vi "Do.vi"(8 "Error In":errorcluster, 10 "Actor in":refnum<class "Actor.lvclass">, 11 "CS++LNAMessage":refnum<class "CS++LNAMessage.lvclass">) -> (0 "Error Out":errorcluster, 2 "Actor out":refnum<class "Actor.lvclass">)   [LabVIEW 2014, in "CS++LNA.lvlib" / "CS++LNAMessage.lvclass"]
doc: "This VI creates the desired message object as class default object. Derives message classes need to override the <b>Parameter to Attribute.vi</b> to parse the variant attributes to the message object attribute.\n\nVI-Parameter Names of corresponding public VI of the derived actor class = Variant Attribute Names\n\n(<B>Filename</B>: Actor Framework.lvlib:Message.lvclass:Do.vi)\n\nDefines what a message does when it is received by an actor. Generally, a message instructs an actor to invoke one of its methods. By default, this method does nothing. A child class must override it to define behavior. Create a child class by using the Actor Framework Message Maker dialog box."
uses:
  CS++LNAMessage.lvclass
  <vilib>/ActorFramework/Actor/Actor.lvclass
  <vilib>/ActorFramework/Message/Message.lvclass
  CS++LNAMessage.lvclass/CS++LNAMessage.ctl
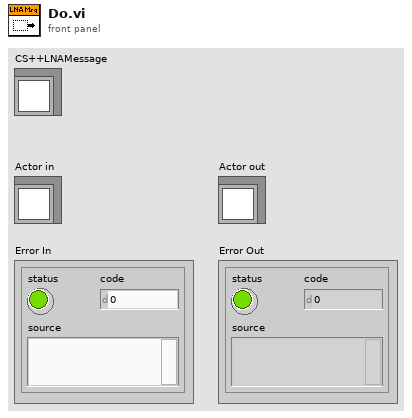
[diagram p1: front panel]
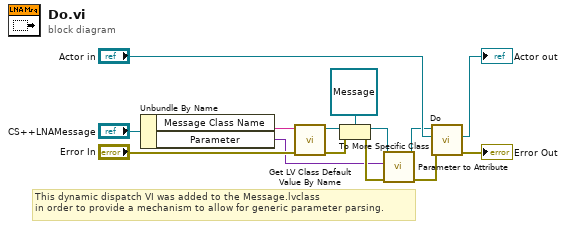
[diagram p0: block diagram]
diagram:
  # "This dynamic dispatch VI was added to the Message.lvclass\nin order to provide a mechanism to allow for generic parameter parsing."
  n1 = Unbundle By Name("CS++LNAMessage") -> ("Message Class Name"=w7:string, "Parameter"=w1:variant)
  n2 = call <vilib>:"Get LV Class Default Value By Name.vi"("error in (no error)"="Error In", "class name"=w7) -> ("error out"=w10:errorcluster, "object"=w9:refnum<class>)  [unwired: 8 in]
  n3 = To More Specific Class(target class=refnum<class "Message.lvclass"> refnum ("Message"), reference=w9, error in=w10) -> (specific class reference=w5:refnum<class "Message.lvclass">, error out=w3:errorcluster)
  n4 = call-dynamic "Parameter to Attribute.vi"("error in (no error)"=w3, "Parameter"=w1, "Message in"=w5) -> ("error out"=w2:errorcluster, "Message out"=w4:refnum<class "Message.lvclass">)  [unwired: 7 in]
  n5 = call-dynamic "Do.vi"("error in (no error)"=w2, "Actor in"="Actor in", "Message"=w4) -> ("error out"=→"Error Out":errorcluster, "Actor out"=→"Actor out":refnum<class "Actor.lvclass">)  [unwired: 7 in]
